vi "PH_GUI.Manager Close.vi"(0 "i ref in":refnum<vi>, 5 "error in":errorcluster) -> (14 "i ref out":refnum<vi>, 19 "error out":errorcluster)   [LabVIEW 2014, in "PH_Common.lvlib"]
doc: "This VI has typically to be set in the destructor of a class. In case of \"Manager File Path\" is not empty or \"N/A\", it writes the current position of the GUI to a xml-file to the place and file name wired."
uses:
  PH_Common.lvlib
  <vilib>/Utility/xml.llb/Write to XML File(string).vi
  CS_Core/CSObj/CSObj.lvlib
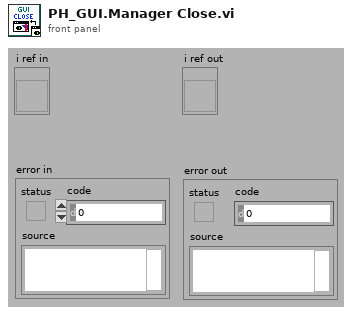
[diagram p1: front panel]
types:
  T1 = typedef "LVRectTypeDef.ctl" = cluster{"Left":i16, "Top":i16, "Right":i16, "Bottom":i16}
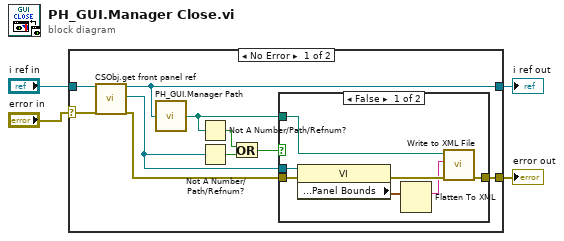
[diagram p0: block diagram]
diagram:
  n1 = case shown="No Error" "error in" {
    selector: "error in" -> [w14 w24]
    tunnel: [w13 w24] -> w4
    tunnel: [w8 w23] -> w3
    tunnel: "i ref in" -> [w12 w23]
    frame No Error {
      n2 = call "CSObj.get front panel ref.vi"("i ref in"=w12, "error in (no error)"=w14) -> ("i ref out"=w8:refnum<vi>, "frontPanelRef"=w10:refnum<vi>, "error out"=w11:errorcluster)  [unwired: 15 in]
      n3 = call "PH_GUI.Manager Path.vi"("i ref in"=w8) -> ("GUI Manager Path"=w9:path)
      n4 = Not A Number/Path/Refnum?(number/path/refnum=w9) -> (NaN/Path/Refnum?=w6:bool)
      n5 = Not A Number/Path/Refnum?(number/path/refnum=w10) -> (NaN/Path/Refnum?=w5:bool)
      n6 = Or(x=w6, y=w5) -> (x .or. y?=w7:bool)
      n7 = case shown="False" w7 {
        tunnel: [w17 w22] -> w13
        tunnel: w11 -> [w21 w22]
        tunnel: w10 -> [w20 _]
        tunnel: w9 -> [w16 _]
        frame False {
          n8 = property class="VI"(reference=w20, error in=w21) -> (error out=w18:errorcluster, "Front Panel Window:Panel Bounds"=w19:T1)  [unwired: 1 out]
          n9 = Flatten To XML(anything=w19) -> (xml string=w15:string)
          n10 = call-poly <vilib>:"Write to XML File.vi"("error in (no error)"=w18, "XML Input"=w15, "XML File Path"=w16) -> ("error out"=w17:errorcluster)  [unwired: 6 in, 2 out]
        }
        frame True {
        }
      }
    }
    frame Error {
    }
  }
  "error out" <- w4
  "i ref out" <- w3
